vi "Reports.Results Chicony CSV Record Data to Test Result V2 JSON.vi"(10 "Data":string[](array[string]), 11 "Header":string[](array[string])) -> (2 "File Name":string, 3 "Test Result V2.0.0":T1={"Type"="TestExec Data", "Version"="2.0.0", "TestEvent"={"ProcessStep"="", "StartTime"="", "EndTime"="", "Mode"="Production", "Operator"="", "Comment"="", "Result"={"State"="", "Code"=0, "Desc"="", "Details"=""}}, "UUTInfo"={"PN"="", "SN"="", "LotNumber"="", "DateCode"="", "AltID"="", "Properties"=[], "Revision"=""}, "Station"={"Name"="", "Location"="", "ConfigID"="", "PCName"="", "Slot"=""}, "TestSequence"={"Name"="", "Setup"=[]}, "ResultData"=[], "DataObjs"=[]})   [LabVIEW 2018]
uses:
  Report.Result State.ctl
  Report.Result Numeric.ctl
  Report.Result DataObject.ctl
  Report.Result Data JSON V2.0.0.ctl
  Report.Result Test Event.ctl
  Report.Result Test Sequence.ctl
  Report.Result Test Station.ctl
  Results/Result XML/TestResult.Facility.ctl
  Results/Result XML/TestResult.HW Item.ctl
  Results/Result XML/TestResult.SW Item.ctl
  Results/Result XML/TestResult.Station Info.ctl
  Results/Result XML/TestResult.Test Run Info.ctl
  Results/Result XML/TestResult.Test Info.ctl
  Results/Result XML/TestResult.Symptom.State.ctl
  Results/Result XML/TestResult.Symptom.ctl
  Results/Result.Measurement and Attribute Item Status.ctl
  Results/Result XML/TestResult.UUT Result.ctl
  Results/Result XML/TestResult.FullResultData.ctl
  Report.Result UUTInfo.ctl
  Time/Time.Format Selector.ctl
  Results/Result.Measurement Item.ctl
  Report.Result Measurement JSON Safe.ctl
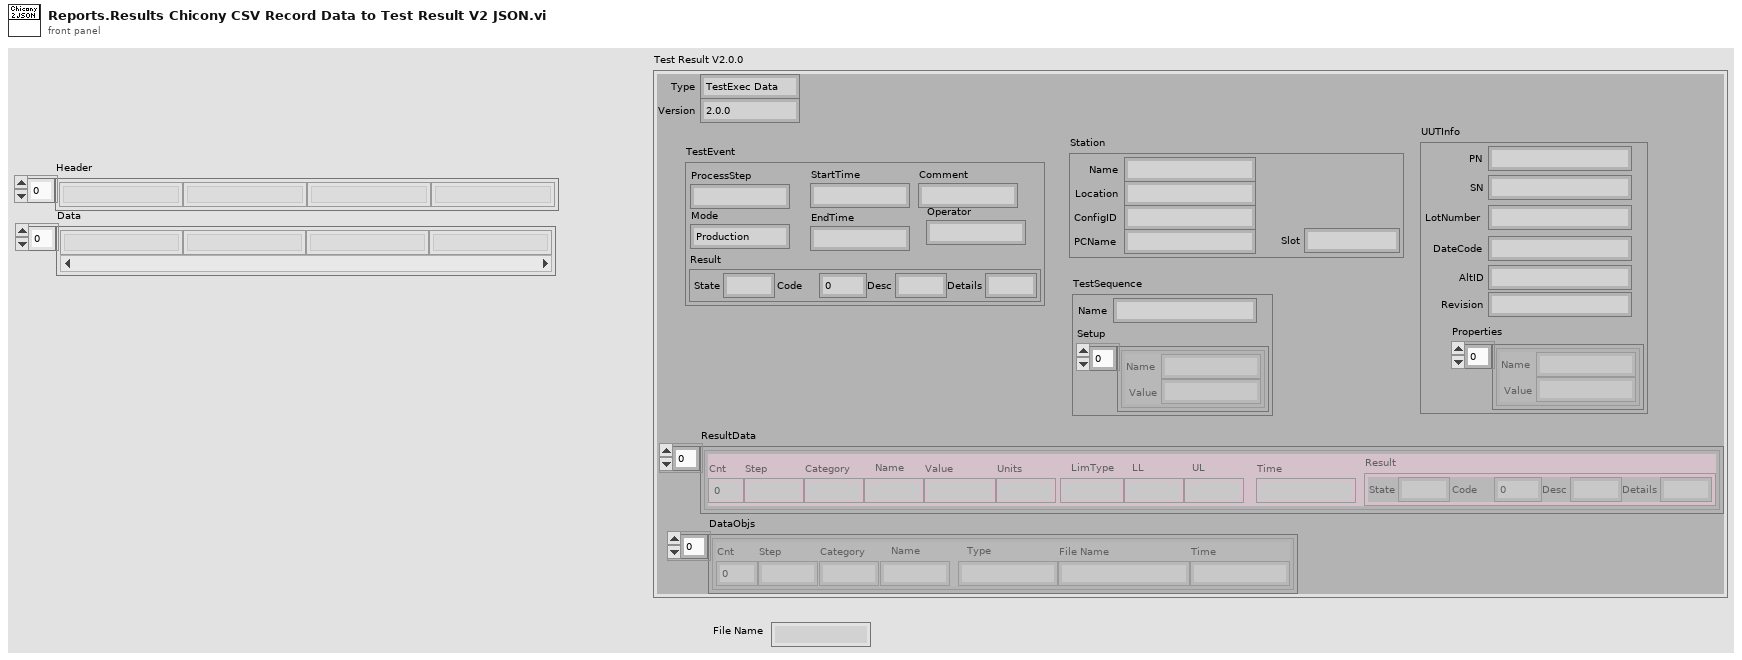
[diagram p1: front panel]
types:
  T1 = typedef "Report.Result Data JSON V2.0.0.ctl" = cluster{"Type":string, "Version":string, "TestEvent":T2, "UUTInfo":T4, "Station":T5, "TestSequence":T6, "ResultData":T7[], "DataObjs":T8[]}
  T2 = typedef "Report.Result Test Event.ctl" = cluster{"ProcessStep":string, "StartTime":string, "EndTime":string, "Mode":string, "Operator":string, "Comment":string, "Result":T3}
  T3 = typedef "Report.Result State.ctl" = cluster{"State":string, "Code":i32, "Desc":string, "Details":string}
  T4 = typedef "Report.Result UUTInfo.ctl" = cluster{"PN":string, "SN":string, "LotNumber":string, "DateCode":string, "AltID":string, "Properties":cluster{"Name":string, "Value":string}[], "Revision":string}
  T5 = typedef "Report.Result Test Station.ctl" = cluster{"Name":string, "Location":string, "ConfigID":string, "PCName":string, "Slot":string}
  T6 = typedef "Report.Result Test Sequence.ctl" = cluster{"Name":string, "Setup":cluster{"Name":string, "Value":string}[]}
  T7 = typedef "Report.Result Measurement JSON Safe.ctl" = cluster{"Cnt":i32, "Step":string, "Category":string, "Name":string, "Value":string, "Units":string, "LimType":string, "LL":string, "UL":string, "Time":string, "Result":T3}
  T8 = typedef "Report.Result DataObject.ctl" = cluster{"Cnt":i32, "Step":string, "Category":string, "Name":string, "Type":string, "File Name":string, "Time":string}
  T9 = typedef "TestResult.FullResultData.ctl" = cluster{"#attributes":cluster{"Version":string}, "Facility":T10, "Station":T11, "Test Run":T14, "Test Sequence":T15, "UUTs":cluster{"UUT":T16[]}}
  T10 = typedef "TestResult.Facility.ctl" = cluster{"Name":string, "Location":string}
  T11 = typedef "TestResult.Station Info.ctl" = cluster{"Name":string, "PN":string, "SN":string, "Rev":string, "PC Name":string, "Location":string, "HW_Config":cluster{"HW_Item":T12[]}, "SW_Config":cluster{"SW_Item":T13[]}}
  T12 = typedef "TestResult.HW Item.ctl" = cluster{"Name":string, "MFG":string, "PN":string, "SN":string, "SW/FW":string, "Note":string, "Cal_ID":string, "Cal_Type":string, "Cal_Due_Date":timestamp, "Cal_Status":string}
  T13 = typedef "TestResult.SW Item.ctl" = cluster{"Name":string, "PN":string, "Version":string, "Note":string}
  T14 = typedef "TestResult.Test Run Info.ctl" = cluster{"Operator":string, "Start Time":timestamp, "Duration(s)":dbl, "Mode":string, "Comment":string, "ProcessStep":string}
  T15 = typedef "TestResult.Test Info.ctl" = cluster{"Name":string, "Config":cluster{"Config_Item":cluster{"Name":string, "Value":string}[]}}
  T16 = typedef "TestResult.UUT Info.ctl" = cluster{"Position":string, "PN":string, "SN":string, "Properties":cluster{"Property":cluster{"Name":string, "Value":string}[]}, "Result":T17, "Measurements":cluster{"Measurement":T19[]}}
  T17 = typedef "TestResult.Symptom.ctl" = cluster{"Result":T18, "Code":i32, "Description":string}
  T18 = typedef "TestResult.Symptom.State.ctl" = enum16{"Pass", "Fail", "Error", "Aborted", "Completed", "Logged"}
  T19 = typedef "Result.Measurement Item.ctl" = cluster{"Cnt":i32, "Step":string, "Category":string, "Name":string, "Value":string, "Units":string, "LimType":string, "LL":string, "UL":string, "Status":T20, "Code":i32, "Desc":string, "Time":timestamp}
  T20 = typedef "Result.Measurement and Attribute Item Status.ctl" = i32
  T21 = typedef "Time.Format Selector.ctl" = enum16{"yyyy/mm/dd HH:MM:S.sss", "yyyy-MM-ddTHH:mm:ss[.mmm]"}
  T22 = typedef "Report.Result Numeric.ctl" = cluster{"Cnt":i32, "Step":string, "Category":string, "Name":string, "Value":dbl, "Units":string, "LimType":string, "LL":dbl, "UL":dbl, "Time":string, "Result":T3}
  T23 = cluster{"Rslt":T1, "Cnt":i32, "Data":string[], "Header":string[], "Start":timestamp}
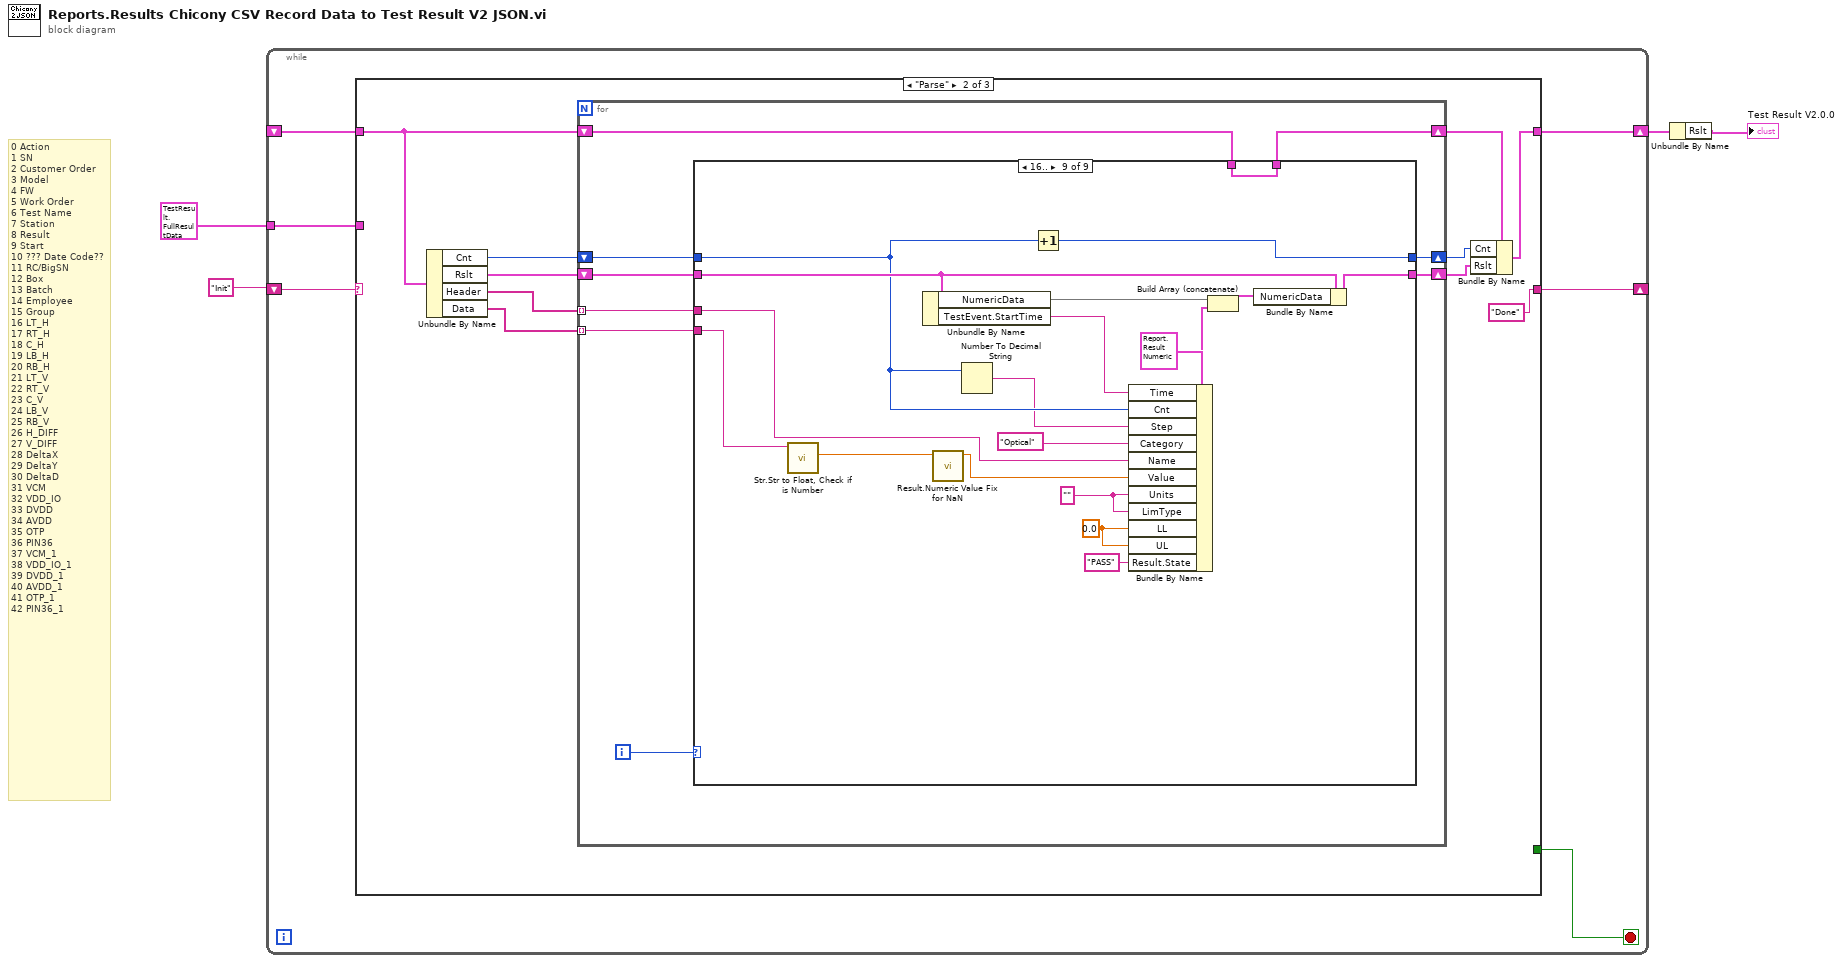
[diagram p0: block diagram]
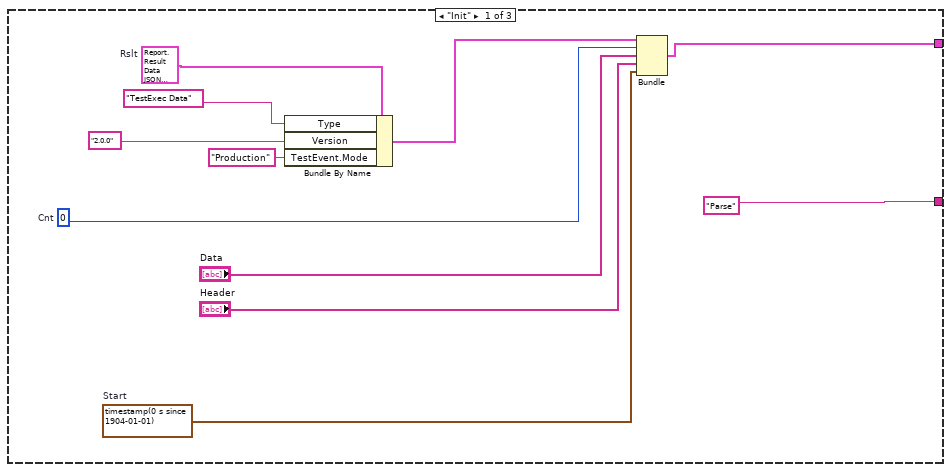
[diagram p2: hidden frame]
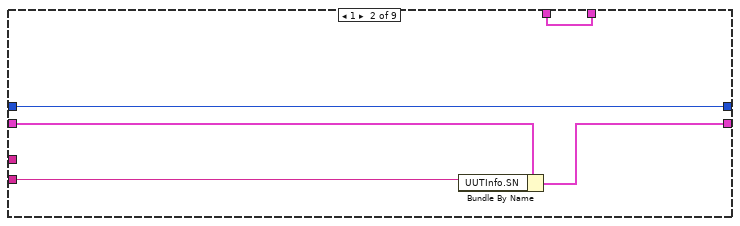
[diagram p4: hidden frame]
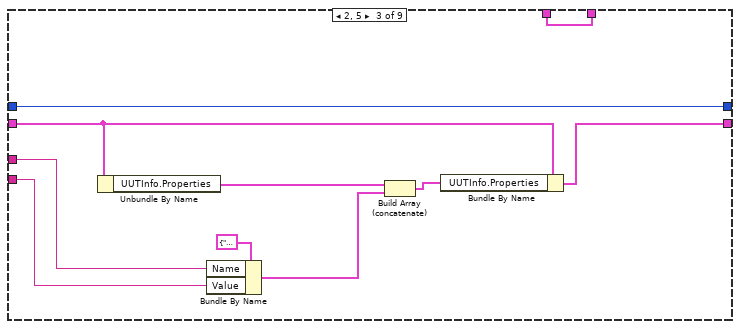
[diagram p5: hidden frame]
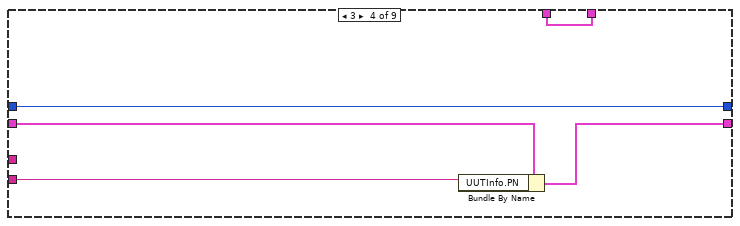
[diagram p6: hidden frame]
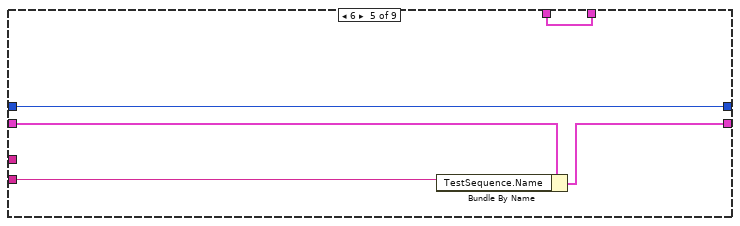
[diagram p7: hidden frame]
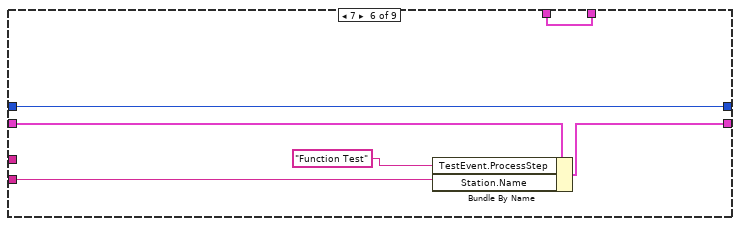
[diagram p8: hidden frame]
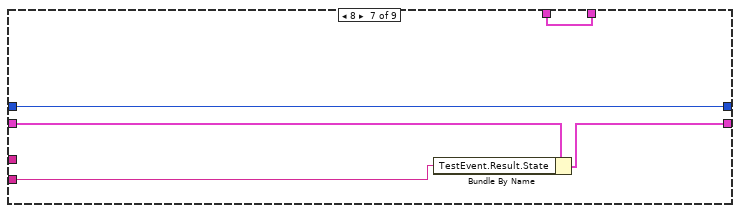
[diagram p9: hidden frame]
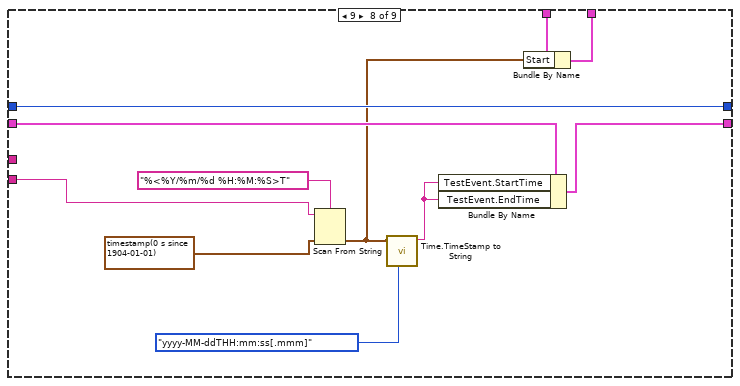
[diagram p10: hidden frame]
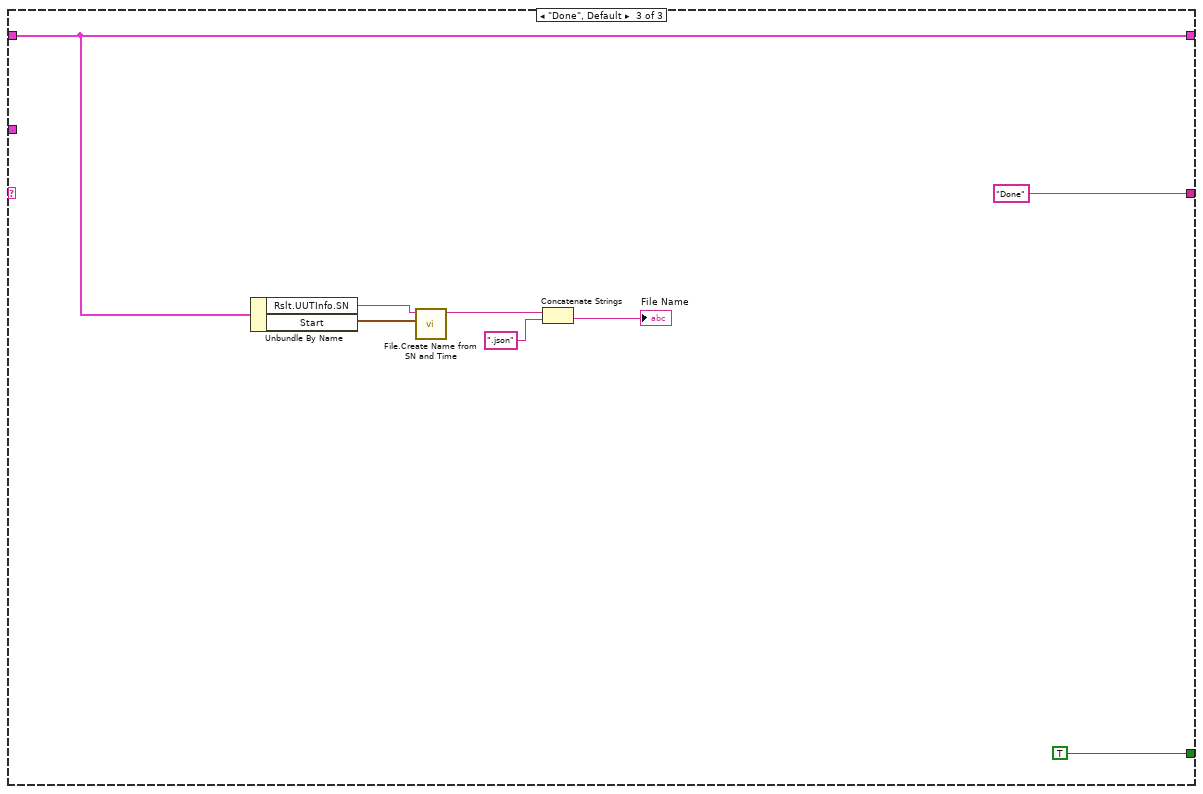
[diagram p11: hidden frame]
diagram:
  # "0\tAction\n1\tSN\n2\tCustomer Order\n3\tModel\n4\tFW\n5\tWork Order\n6\tTest Name\n7\tStation\n8\tResult\n9\tStart\n10\t??? Date Code??\n11\tRC/BigSN\n12\tBox\n13\tBatch\n14\tEmployee\n15\tGroup\n16\tLT_H\n17\tRT_H\n18\tC_H\n19\tLB_H\n20\tRB_H\n21\tLT_V\n22\tRT_V\n23\tC_V\n24\tLB_V\n25\tRB_V\n26\tH_DIFF\n27\tV_DIFF\n28\tDeltaX\n29\tDeltaY\n30\tDeltaD\n31\tVCM\n32\tVDD_IO\n33\tDVDD\n34\tAVDD\n35\tOTP\n36\tPIN36\n37\tVCM_1\n38\tVDD_IO_1\n39\tDVDD_1\n40\tAVDD_1\n41\tOTP_1\n42\tPIN36_1"
  n1 = while {
    shift-right: [w5] -> w2
    shift-left: _ -> [w10]
    shift-right: [w7] -> _
    shift-left: "Init" -> [w8]
    tunnel: T9 {"#attributes"={"Version"="MTE_1.0.0"}, "Facility"={"Name"="", "Location"=""}, "Station"={"Name"="", "PN"="", "SN"="", "Rev"="", "PC Name"="", "Location"="", "HW_Config"={"HW_Item"=[]}, "SW_Config"={"SW_Item"=[]}}, "Test Run"={"Operator"="", "Start Time"=timestamp(0 s since 1904-01-01), "Duration(s)"=0.0, "Mode"="", "Comment"="", "ProcessStep"=""}, "Test Sequence"={"Name"="", "Config"={"Config_Item"=[]}}, "UUTs"={"UUT"=[]}} ("Test Result In") -> [w6]
    stop <- w9 stop-if-true
    n2 = case shown="\"Parse\"" w8 {
      tunnel: w10 -> [_ w23 w115]
      tunnel: [w15 w26 w115] -> w5
      tunnel: [_ _ TRUE] -> w9
      tunnel: ["Parse" ("Version") "Done" ("Version") "Done"] -> w7
      tunnel: w6 -> [_ _ _]
      frame "Init" {
        w12 = timestamp(0 s since 1904-01-01)  # Start
        w16 = 0  # Cnt
        w19 = T1 {"Type"="Test Data", "Version"="1.0.0", "TestEvent"={"ProcessStep"="", "StartTime"="", "EndTime"="", "Mode"="", "Operator"="", "Comment"="", "Result"={"State"="", "Code"=0, "Desc"="", "Details"=""}}, "UUTInfo"={"PN"="", "SN"="", "LotNumber"="", "DateCode"="", "AltID"="", "Properties"=[], "Revision"=""}, "Station"={"Name"="", "Location"="", "ConfigID"="", "PCName"="", "Slot"=""}, "TestSequence"={"Name"="", "Setup"=[]}, "ResultData"=[], "DataObjs"=[]}  # Rslt
        n3 = Bundle By Name(cluster=w19, "Type"="TestExec Data", "Version"="2.0.0", "TestEvent.Mode"="Production") -> (w17:T1)
        n4 = Bundle("Rslt"=w17, "Cnt"=w16, "Data"="Data", "Header"="Header", "Start"=w12) -> (w15:T23)  [unwired: 1 in]
      }
      frame "Parse" {
        n5 = Unbundle By Name(w23) -> ("Cnt"=w29:i32, "Rslt"=w31:T1, "Header"=w30:string[], "Data"=w24:string[])
        n6 = for {
          shift-right: [w39] -> w28
          shift-left: w31 -> [w40]
          tunnel: w30 -> [w34] mode=indexing
          shift-right: [w37] -> w27
          shift-left: w29 -> [w38]
          tunnel: w24 -> [w35] mode=indexing
          shift-right: [w32] -> w22
          shift-left: w23 -> [w33]
          i -> [w36]
          n7 = case shown="16.." w36 {
            tunnel: w40 -> [w42 w48 w56 w63 w68 w74 w79 w90 w109]
            tunnel: [w42 w47 w58 w62 w67 w73 w78 w89 w108] -> w39
            tunnel: w38 -> [w43 w46 w57 w61 w66 w72 w77 w88 w92]
            tunnel: [w43 w46 w57 w61 w66 w72 w77 w88 w107] -> w37
            tunnel: w35 -> [_ w45 w50 w60 w65 w71 w76 w85 w98]
            tunnel: w34 -> [_ _ w51 _ _ _ _ _ w97]
            tunnel: w33 -> [w41 w44 w49 w59 w64 w69 w75 w82 w94]
            tunnel: [w41 w44 w49 w59 w64 w69 w75 w80 w94] -> w32
            frame 0, Default {
              # "Skip"
            }
            frame 1 {
              n8 = Bundle By Name(cluster=w48, "UUTInfo.SN"=w45) -> (w47:T1)
            }
            frame 2, 5 {
              n9 = Unbundle By Name(w56) -> ("UUTInfo.Properties"=w55:cluster{"Name":string, "Value":string}[])
              n10 = Bundle By Name(cluster=cluster{"Name":string, "Value":string} {"Name"="", "Value"=""} ("Setup"), "Name"=w51, "Value"=w50) -> (w52:cluster{"Name":string, "Value":string})
              n11 = Build Array (concatenate)(w55, w52) -> (w54:cluster{"Name":string, "Value":string}[])
              n12 = Bundle By Name(cluster=w56, "UUTInfo.Properties"=w54) -> (w58:T1)
            }
            frame 3 {
              n13 = Bundle By Name(cluster=w63, "UUTInfo.PN"=w60) -> (w62:T1)
            }
            frame 6 {
              n14 = Bundle By Name(cluster=w68, "TestSequence.Name"=w65) -> (w67:T1)
            }
            frame 7 {
              n15 = Bundle By Name(cluster=w74, "TestEvent.ProcessStep"="Function Test", "Station.Name"=w71) -> (w73:T1)
            }
            frame 8 {
              n16 = Bundle By Name(cluster=w79, "TestEvent.Result.State"=w76) -> (w78:T1)
            }
            frame 9 {
              n17 = Scan From String(format string="%<%Y/%m/%d %H:%M:%S>T", input string=w85, default 1=timestamp(0 s since 1904-01-01)) -> (output 1=w81:timestamp)  [unwired: 2 in, 3 out]
              n18 = call "Time.TimeStamp to String.vi"("TimeFormat"=Time.Format_Selector."yyyy-MM-ddTHH:mm:ss[.mmm]", "Time Stamp in"=w81) -> ("Time String Out"=w84:string)  [unwired: 9 in]
              n19 = Bundle By Name(cluster=w90, "TestEvent.StartTime"=w84, "TestEvent.EndTime"=w84) -> (w89:T1)
              n20 = Bundle By Name(cluster=w82, "Start"=w81) -> (w80:T23)
            }
            frame 16.. {
              w95 = 0.0 ("LL")
              w96 = "" ("Units")
              n21 = call "Str.Str to Float, Check if is Number.vi"("Value In"=w98) -> ("Num Out"=w106:dbl)  [unwired: 8 in, 2 out]
              n22 = Unbundle By Name(w109) -> ("NumericData"=w105, "TestEvent.StartTime"=w100:string)
              n23 = call "Result.Numeric Value Fix for NaN.vi"("Numeric"=w106) -> ("Numeric Out"=w101:dbl)  [unwired: 10 in]
              n24 = Number To Decimal String(number=w92) -> (decimal integer string=w91:string)  [unwired: 1 in]
              n25 = Increment(x=w92) -> (x+1=w107:i32)
              n26 = Bundle By Name(cluster=T22 {"Cnt"=0, "Step"="", "Category"="", "Name"="", "Value"=0.0, "Units"="", "LimType"="", "LL"=0.0, "UL"=0.0, "Time"="", "Result"={"State"="", "Code"=0, "Desc"="", "Details"=""}} ("Numeric"), "Time"=w100, "Cnt"=w92, "Step"=w91, "Category"="Optical" ("Step"), "Name"=w97, "Value"=w101, "Units"=w96, "LimType"=w96, "LL"=w95, "UL"=w95, "Result.State"="PASS") -> (w102:T22)
              n27 = Build Array (concatenate)(w105, w102) -> (w104:T22[])
              n28 = Bundle By Name(cluster=w109, "NumericData"=w104) -> (w108:T1)
            }
          }
        }
        n29 = Bundle By Name(cluster=w22, "Cnt"=w27, "Rslt"=w28) -> (w26:T23)
      }
      frame "Done", Default {
        n30 = Unbundle By Name(w115) -> ("Rslt.UUTInfo.SN"=w114:string, "Start"=w113:timestamp)
        n31 = call "File.Create Name from SN and Time.vi"("StartTime"=w113, "SN"=w114) -> ("SN_Time"=w112:string)  [unwired: 9 in]
        n32 = Concatenate Strings(w112, ".json" ("string")) -> (→"File Name":string)
      }
    }
  }
  n33 = Unbundle By Name(w2) -> ("Rslt"=→"Test Result V2.0.0":T1)
